vi "Set State.vi"(8 "error in (no error)":errorcluster, 10 "State":T1, 11 "VISA Client in":refnum<class "Serial Client.lvclass">) -> (0 "error out":errorcluster, 3 "VISA Client out":refnum<class "Serial Client.lvclass">)   [LabVIEW 2020, in "Stream-Serial.lvlib" / "Serial Client.lvclass"]
uses:
  Serial Client.lvclass
  Connection State.ctl
  Serial Client.lvclass/Serial Client.ctl
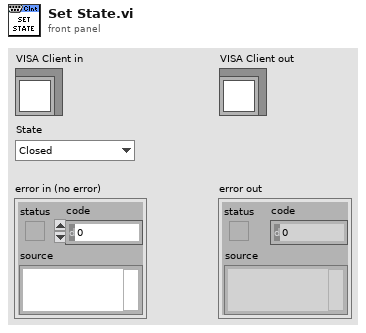
[diagram p1: front panel]
types:
  T1 = typedef "Stream-Serial.lvlib/Serial Client.lvclass/Connection State.ctl" = enum16{"Closed", "Idle", "Connecting", "Connected", "Shutdown"}
  T2 = typedef "Stream-Serial.lvlib/Serial Client.lvclass/Ref Data.ctl" = cluster{"VISA Stream":refnum<class "Serial Stream.lvclass">, "State":T1, "Client Loop":refnum<vi>, "VISA Resource":refnum<visa-resource-name>}
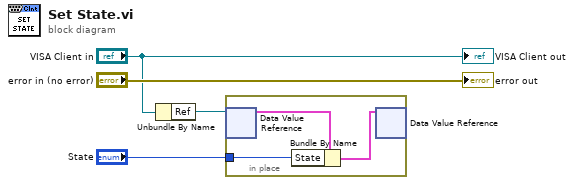
[diagram p0: block diagram]
diagram:
  n1 = Unbundle By Name("VISA Client in") -> ("Ref"=w3:refnum<data-value>)
  n2 = in-place {
    in-place-border: "State" -> [w5]
    n3 = in-place-dvr #1(w3) -> (w7:T2)  [unwired: 1 out]
    n4 = Bundle By Name(cluster=w7, "State"=w5) -> (w6:T2)
    n5 = in-place-dvr #1(w6) -> ()  [unwired: 2 out]
  }
  "error out" <- "error in (no error)"
  "VISA Client out" <- "VISA Client in"
